vi "NewAndLoad.vi"(0 "EpiWrapper in":refnum<class "EpiWrapper.lvclass">, 1 "StartLotTraveler":T1, 2 "Command":T2=enum."INIT", 3 "error in (no error)":errorcluster, 4 "menu reference":refnum<k9>) -> (5 "EpiWrapper out":refnum<class "EpiWrapper.lvclass">, 6 "Message":string, 7 "error out":errorcluster)   [LabVIEW 2012, in "EpiWrapper.lvclass"]
uses:
  EpiWrapper.lvclass
  Controls/TestType.ctl
  Controls/Command_Enum.ctl
  Controls/StartLotTraveler.ctl
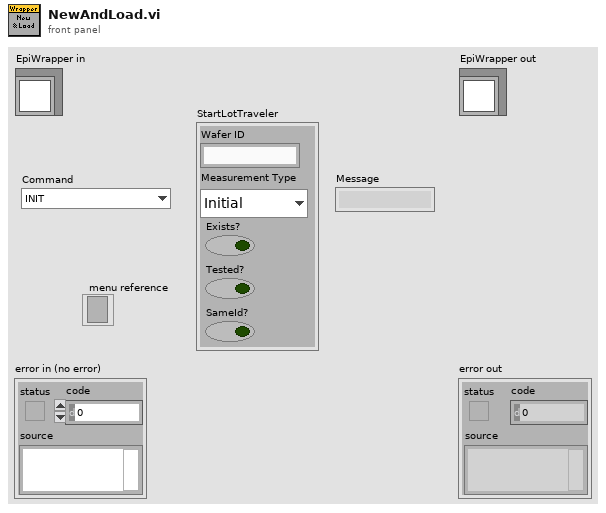
[diagram p1: front panel]
types:
  T1 = typedef "StartLotTraveler.ctl" = cluster{"Wafer ID":string, "Measurement Type":enum16{"Initial", "Final"}, "Exists?":bool, "Tested?":bool, "SameId?":bool}
  T2 = typedef "Command_Enum.ctl" = enum16{"SPECTRUMCAPTURE", "INSITUMEASURE", "RESETCONFIG", "OPENCONFIG", "RESET", "INIT", "LOAD", "MEASURE", "NEW", "SAVE", "UPDATE_INT", "SWAP_MODE", "UPDATE_ACQ", "MARK_MAP_SELECT", "MARK_MAP", "EXIT", "CANCEL"}
  T3 = typedef "TestType.ctl" = string
  T4 = enum8{"Enabled", "Disabled", "Disabled and Grayed Out"}
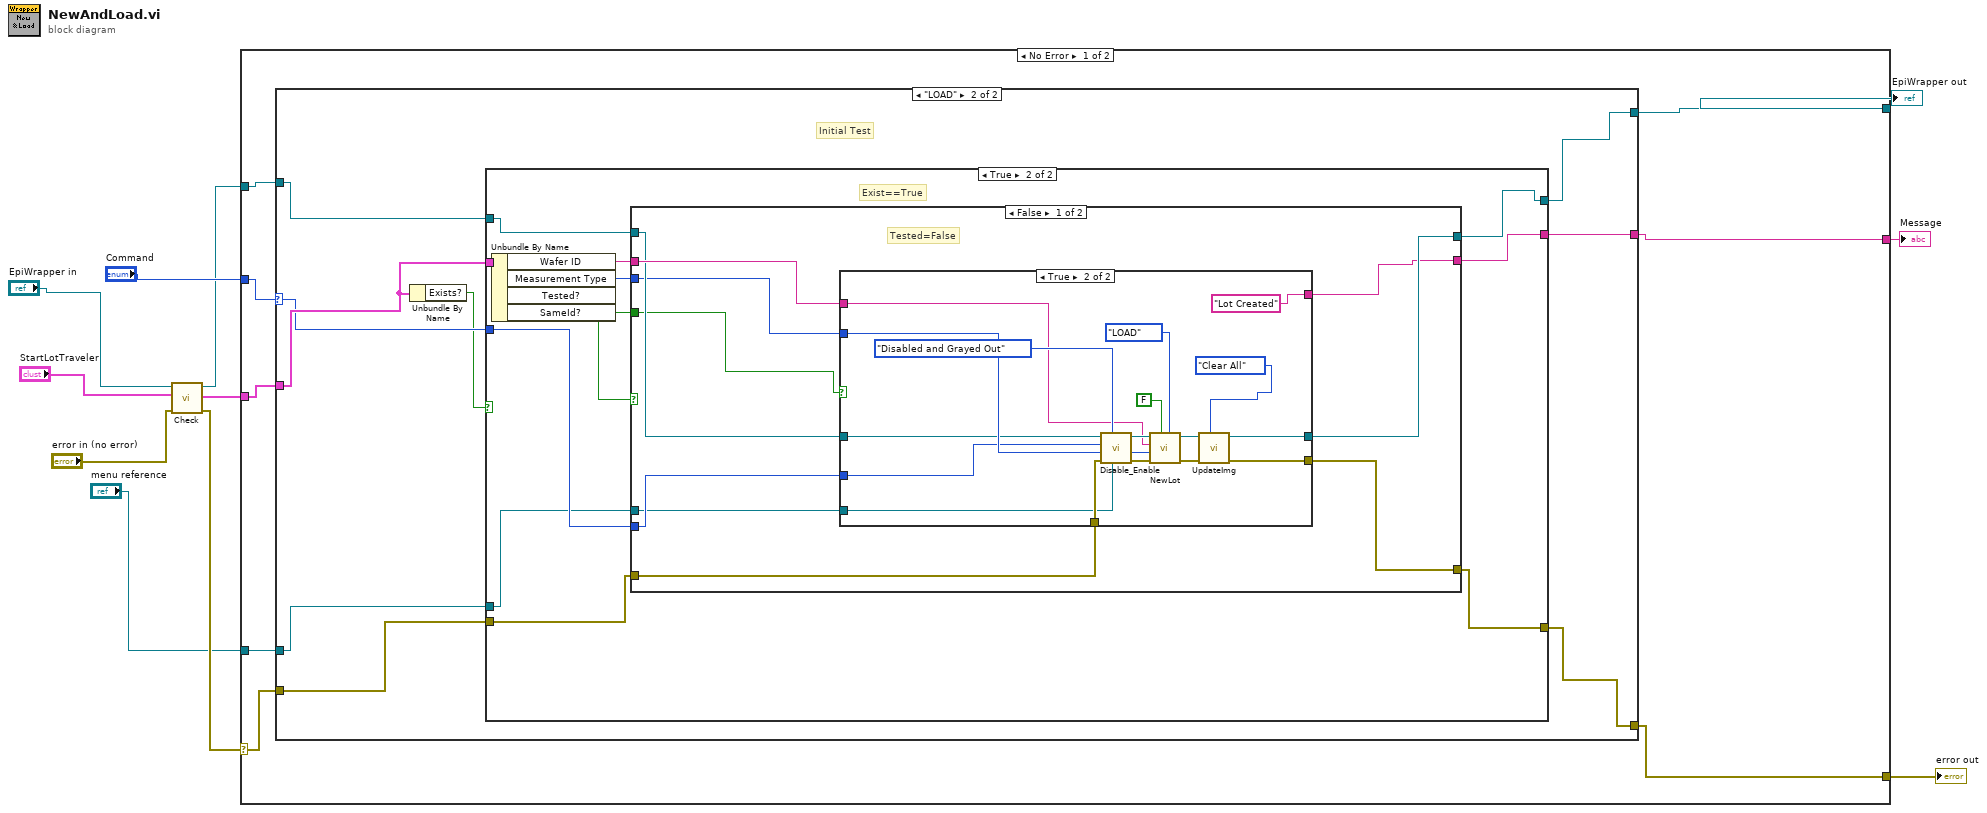
[diagram p0: block diagram]
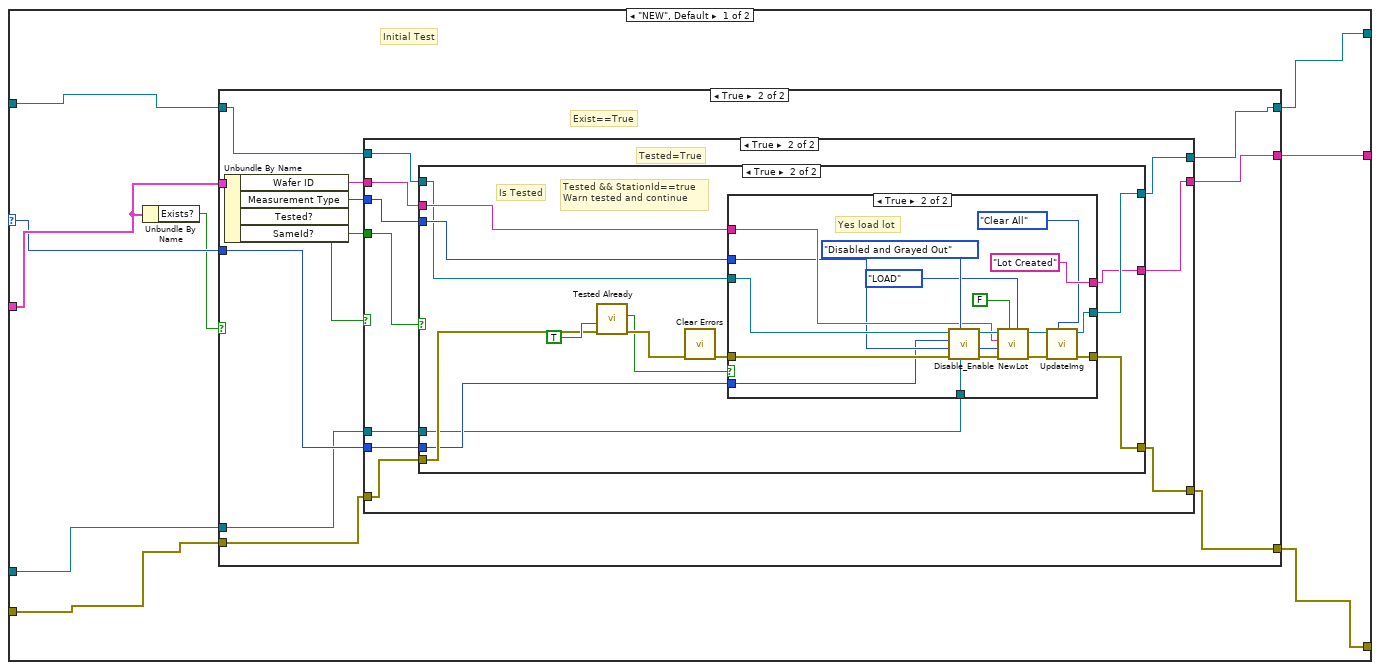
[diagram p2: hidden frame]
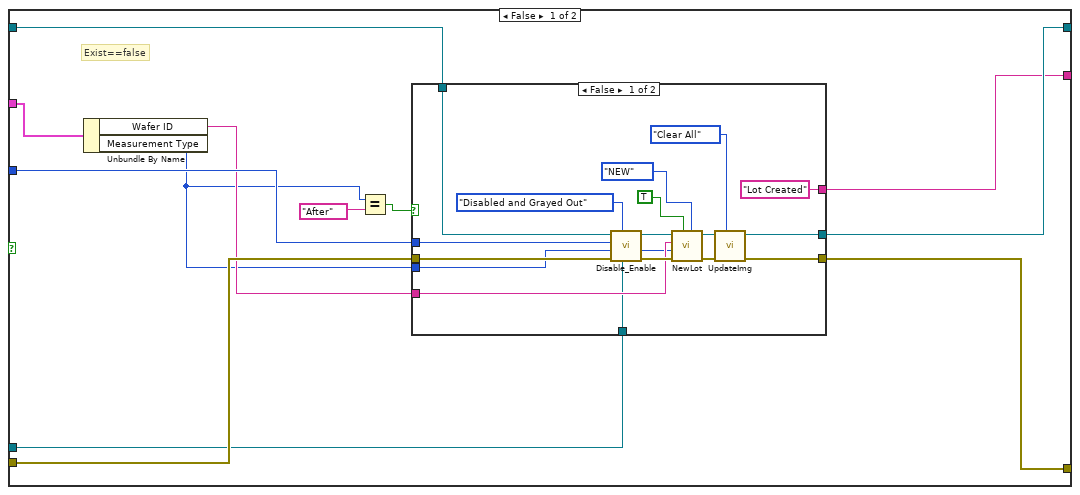
[diagram p3: hidden frame]
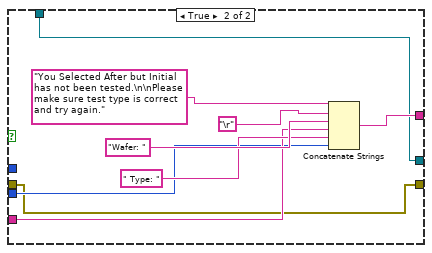
[diagram p4: hidden frame]
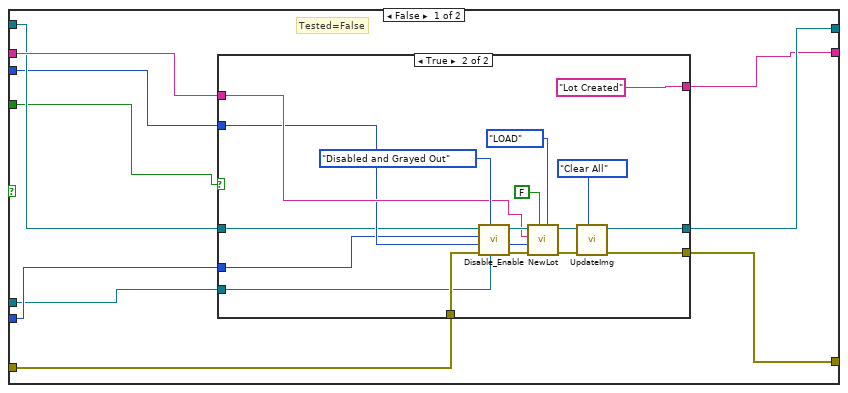
[diagram p5: hidden frame]
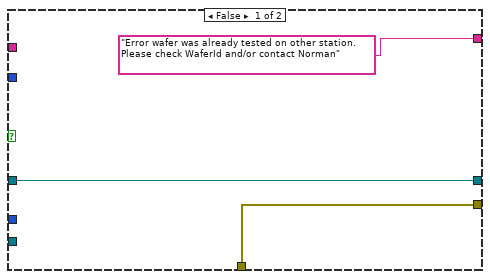
[diagram p6: hidden frame]
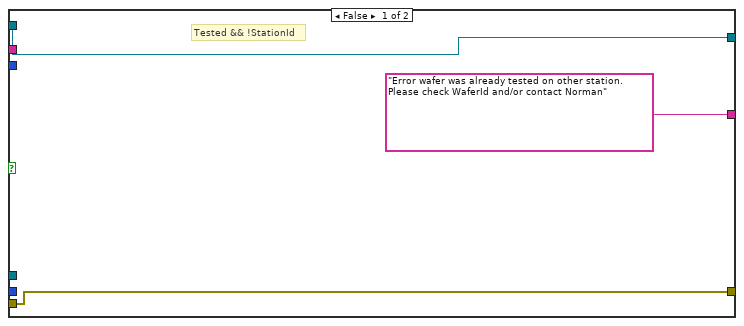
[diagram p7: hidden frame]
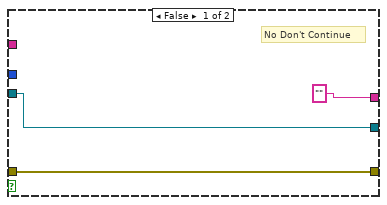
[diagram p8: hidden frame]
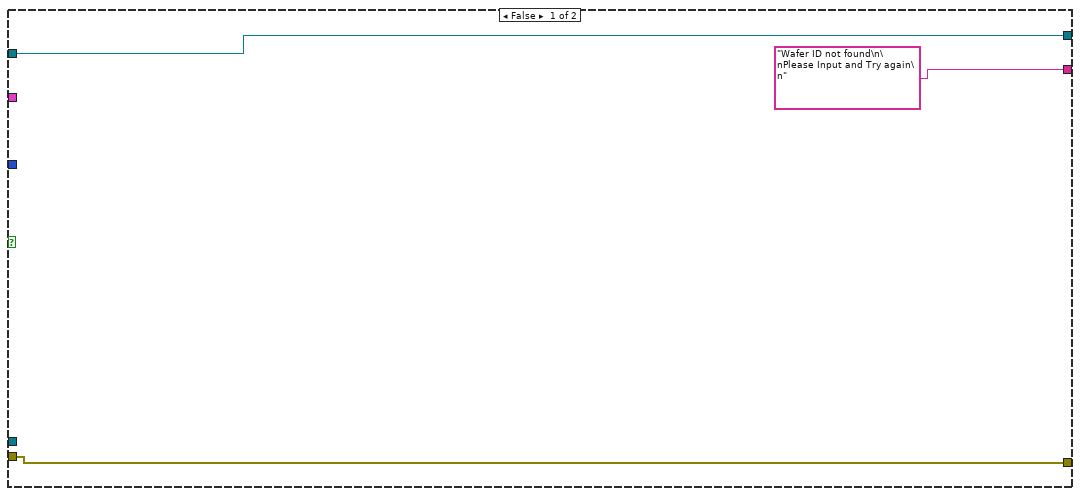
[diagram p9: hidden frame]
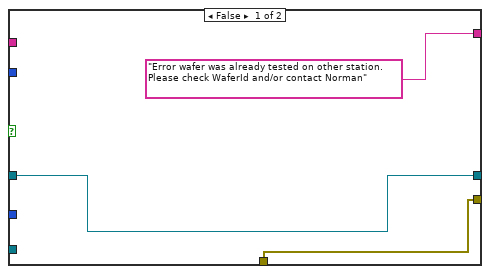
[diagram p10: hidden frame]
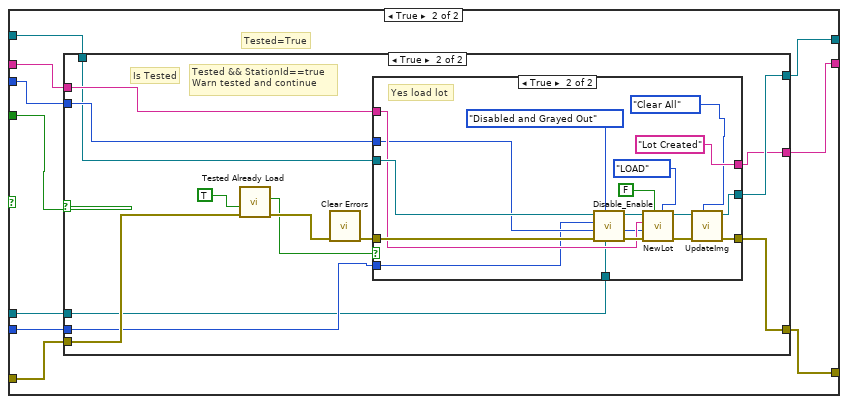
[diagram p11: hidden frame]
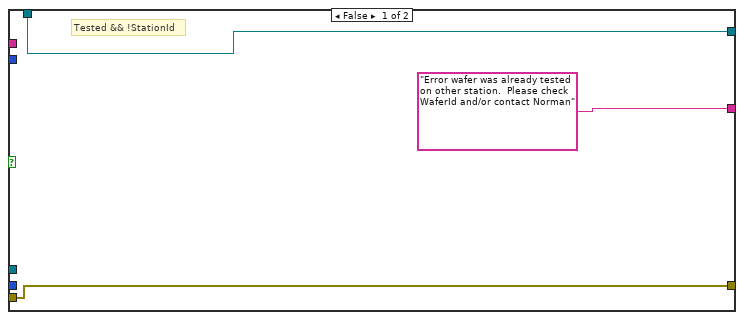
[diagram p12: hidden frame]
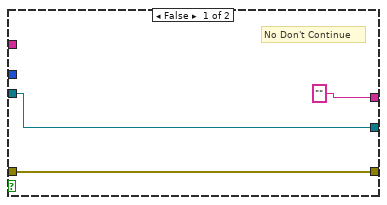
[diagram p13: hidden frame]
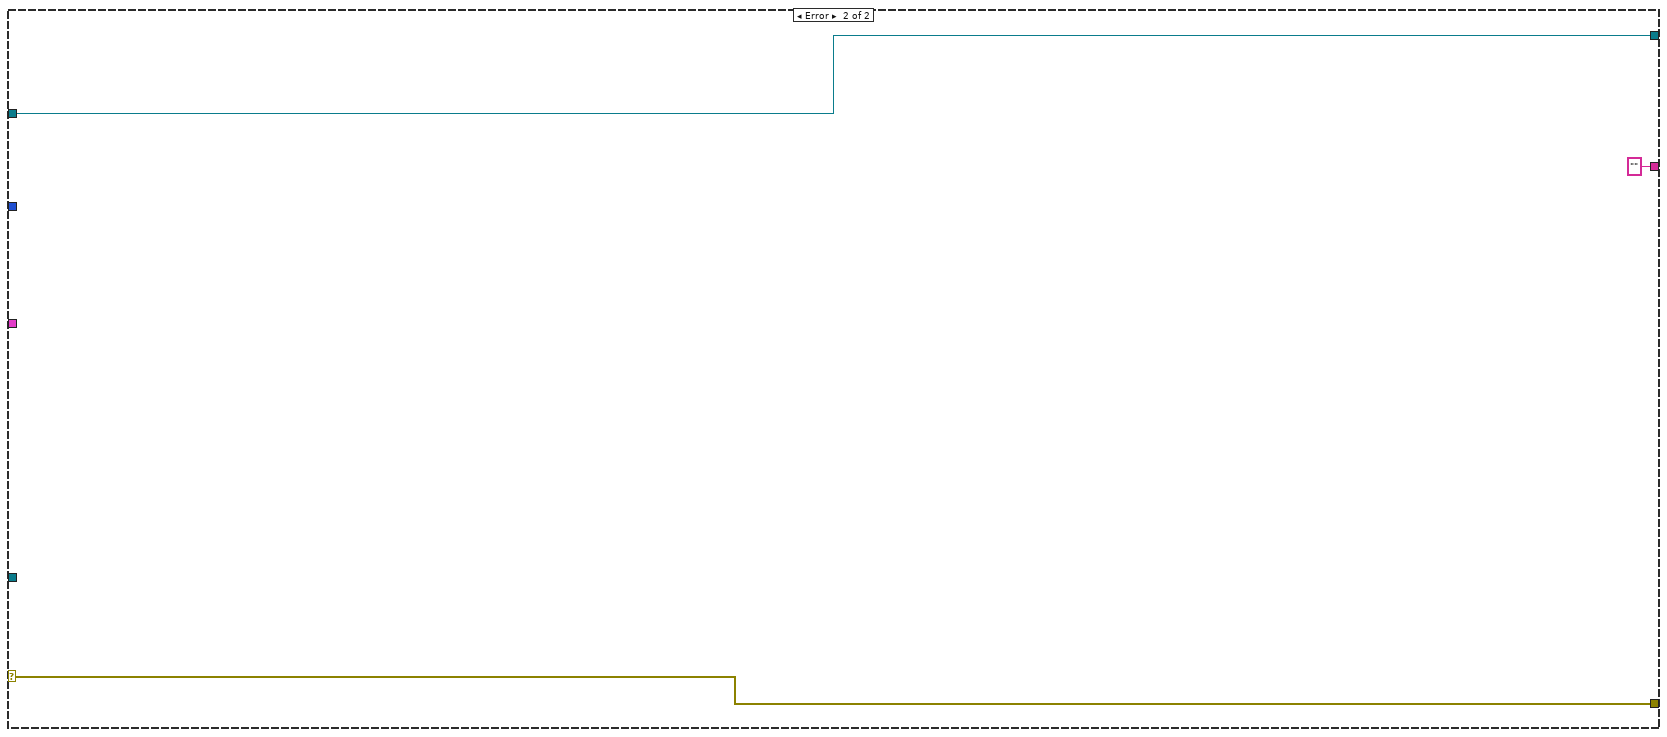
[diagram p14: hidden frame]
diagram:
  n1 = call-dynamic "Check.vi"("error in (no error)"="error in (no error)", "StartLotTraveler In"="StartLotTraveler", "EpiWrapper in"="EpiWrapper in") -> ("error out"=w8:errorcluster, "StartLotTraveler Out"=w7:T1, "EpiWrapper out"=w2:refnum<class "EpiWrapper.lvclass">)  [unwired: 6 in]
  n2 = case shown="No Error" w8 {
    selector: w8 -> [w16 w257]
    tunnel: [w12 w257] -> w11
    tunnel: [w15 w256] -> w10
    tunnel: w2 -> [w17 w256]
    tunnel: w7 -> [w18 _]
    tunnel: "Command" -> [w19 _]
    tunnel: "menu reference" -> [w14 _]
    tunnel: [w13 "" ("x")] -> w1
    frame No Error {
      n3 = case shown="\"LOAD\"" w19 {
        selector: w19 -> [w26 w161]
        tunnel: w18 -> [w28 w163]
        tunnel: w17 -> [w27 w162]
        tunnel: w16 -> [w25 w160]
        tunnel: [w24 w159] -> w15
        tunnel: [w23 w158] -> w12
        tunnel: w14 -> [w22 w157]
        tunnel: [w21 w156] -> w13
        frame "NEW", Default {
          # "Initial Test"
          n4 = Unbundle By Name(w28) -> ("Exists?"=w20:bool)
          n5 = case shown="True" w20 {
            tunnel: w27 -> [w40 w73]
            tunnel: w26 -> [w39 w71]
            tunnel: w25 -> [w38 w72]
            tunnel: w28 -> [w37 w78]
            tunnel: [w35 w68] -> w24
            tunnel: [w34 w69] -> w23
            tunnel: w22 -> [w33 w70]
            tunnel: [w29 w67] -> w21
            frame False {
              # "Exist==false"
              n6 = Unbundle By Name(w37) -> ("Wafer ID"=w36:string, "Measurement Type"=w31:enum16{"Initial", "Final"})
              n7 = Equal?(x=w31, y=T3 "After") -> (x = y?=w30:bool)
              n8 = case shown="False" w30 {
                tunnel: w40 -> [w57 w58]
                tunnel: w39 -> [w56 _]
                tunnel: w38 -> [w55 w59]
                tunnel: w36 -> [w47 w61]
                tunnel: w31 -> [w46 w60]
                tunnel: [w45 w58] -> w35
                tunnel: [w44 w59] -> w34
                tunnel: w33 -> [w43 _]
                tunnel: ["Lot Created" w62] -> w29
                frame False {
                  n9 = call-dynamic "Disable_Enable.vi"("menu reference"=w43, "Disabled"=T4."Disabled and Grayed Out", "error in (no error)"=w55, "Command"=w56, "EpiWrapper in"=w57) -> ("error out"=w51:errorcluster, "EpiWrapper out"=w53:refnum<class "EpiWrapper.lvclass">)  [unwired: 5 in]
                  n10 = call-dynamic "NewLot.vi"("Enum"=enum16{"LOAD", "NEW"}."NEW", "Create Entry?"=TRUE, "error in (no error)"=w51, "Test"=w46, "Wafer ID"=w47, "FrontPanelData in"=w53) -> ("error out"=w52:errorcluster, "FrontPanelData out"=w54:refnum<class "EpiWrapper.lvclass">)  [unwired: 3 in, 1 out]
                  n11 = call-dynamic "UpdateImg.vi"("Enum"=enum16{"Remove", "Mark", "Clear All"}."Clear All", "error in (no error)"=w52, "EpiWrapper in"=w54) -> ("error out"=w44:errorcluster, "EpiWrapper out"=w45:refnum<class "EpiWrapper.lvclass">)  [unwired: 7 in]
                }
                frame True {
                  n12 = Concatenate Strings("You Selected After but Initial has not been tested.\n\nPlease make sure test type is correct and try again.", "\r", "Wafer: " ("string"), w61, " Type: " ("string"), w60) -> (w62:string)
                }
              }
            }
            frame True {
              # "Exist==True"
              n13 = Unbundle By Name(w78) -> ("Wafer ID"=w75:string, "Measurement Type"=w74:enum16{"Initial", "Final"}, "Tested?"=w77:bool, "SameId?"=w76:bool)
              n14 = case shown="True" w77 {
                tunnel: w76 -> [w79 w118]
                tunnel: w75 -> [w88 w117]
                tunnel: w74 -> [w80 w116]
                tunnel: w73 -> [w87 w115]
                tunnel: w72 -> [w85 w114]
                tunnel: w71 -> [w86 w113]
                tunnel: w70 -> [w84 w112]
                tunnel: [w83 w111] -> w69
                tunnel: [w82 w110] -> w68
                tunnel: [w81 w109] -> w67
                frame False {
                  # "Tested=False"
                  n15 = case shown="True" w79 {
                    tunnel: w88 -> [_ w101]
                    tunnel: w80 -> [_ w100]
                    tunnel: w87 -> [w90 w99]
                    tunnel: w86 -> [_ w98]
                    tunnel: w85 -> [w91 w97]
                    tunnel: w84 -> [_ w96]
                    tunnel: [w91 w95] -> w83
                    tunnel: [w90 w94] -> w82
                    tunnel: ["Error wafer was already tested on other station.  Please check WaferId and/or contact Norman" "Lot Created" ("x")] -> w81
                    frame False {
                    }
                    frame True {
                      n16 = call-dynamic "Disable_Enable.vi"("menu reference"=w96, "Disabled"=T4."Disabled and Grayed Out", "error in (no error)"=w97, "Command"=w98, "EpiWrapper in"=w99) -> ("error out"=w107:errorcluster, "EpiWrapper out"=w105:refnum<class "EpiWrapper.lvclass">)  [unwired: 5 in]
                      n17 = call-dynamic "NewLot.vi"("Enum"=enum16{"LOAD", "NEW"}."LOAD", "Create Entry?"=FALSE, "error in (no error)"=w107, "Test"=w100, "Wafer ID"=w101, "FrontPanelData in"=w105) -> ("error out"=w106:errorcluster, "FrontPanelData out"=w104:refnum<class "EpiWrapper.lvclass">)  [unwired: 3 in, 1 out]
                      n18 = call-dynamic "UpdateImg.vi"("Enum"=enum16{"Remove", "Mark", "Clear All"}."Clear All", "error in (no error)"=w106, "EpiWrapper in"=w104) -> ("error out"=w95:errorcluster, "EpiWrapper out"=w94:refnum<class "EpiWrapper.lvclass">)  [unwired: 7 in]
                    }
                  }
                }
                frame True {
                  # "Tested=True"
                  n19 = case shown="True" w118 {
                    tunnel: w117 -> [_ w130]
                    tunnel: w116 -> [_ w129]
                    tunnel: w115 -> [w119 w128]
                    tunnel: w114 -> [w120 w127]
                    tunnel: w113 -> [_ w126]
                    tunnel: w112 -> [_ w125]
                    tunnel: [w120 w124] -> w111
                    tunnel: [w119 w123] -> w110
                    tunnel: ["Error wafer was already tested on other station.  Please check WaferId and/or contact Norman" w122] -> w109
                    frame False {
                      # "Tested && !StationId"
                    }
                    frame True {
                      # "Is Tested"
                      # "Tested && StationId==true\nWarn tested and continue"
                      n20 = call "Tested Already"("error in (no error)"=w127, "Enable"=TRUE) -> ("error out"=w134:errorcluster, "Continue"=w133:bool)  [unwired: 8 in]
                      n21 = call <vilib>:"Clear Errors.vi"("error in (no error)"=w134) -> ("error out"=w131:errorcluster)  [unwired: 6 in]
                      n22 = case shown="True" w133 {
                        tunnel: w131 -> [w137 w153]
                        tunnel: [w137 w150] -> w124
                        tunnel: w128 -> [w136 w146]
                        tunnel: [w136 w145] -> w123
                        tunnel: w130 -> [_ w143]
                        tunnel: w129 -> [_ w142]
                        tunnel: w126 -> [_ w141]
                        tunnel: ["" "Lot Created"] -> w122
                        tunnel: w125 -> [_ w139]
                        frame False {
                          # "No Don't Continue"
                        }
                        frame True {
                          # "Yes load lot"
                          n23 = call-dynamic "Disable_Enable.vi"("menu reference"=w139, "Disabled"=T4."Disabled and Grayed Out", "error in (no error)"=w153, "Command"=w141, "EpiWrapper in"=w146) -> ("error out"=w152:errorcluster, "EpiWrapper out"=w147:refnum<class "EpiWrapper.lvclass">)  [unwired: 5 in]
                          n24 = call-dynamic "NewLot.vi"("Enum"=enum16{"LOAD", "NEW"}."LOAD", "Create Entry?"=FALSE, "error in (no error)"=w152, "Test"=w142, "Wafer ID"=w143, "FrontPanelData in"=w147) -> ("error out"=w151:errorcluster, "FrontPanelData out"=w148:refnum<class "EpiWrapper.lvclass">)  [unwired: 3 in, 1 out]
                          n25 = call-dynamic "UpdateImg.vi"("Enum"=enum16{"Remove", "Mark", "Clear All"}."Clear All", "error in (no error)"=w151, "EpiWrapper in"=w148) -> ("error out"=w150:errorcluster, "EpiWrapper out"=w145:refnum<class "EpiWrapper.lvclass">)  [unwired: 7 in]
                        }
                      }
                    }
                  }
                }
              }
            }
          }
        }
        frame "LOAD" {
          # "Initial Test"
          n26 = Unbundle By Name(w163) -> ("Exists?"=w155:bool)
          n27 = case shown="True" w155 {
            tunnel: w162 -> [w165 w173]
            tunnel: w161 -> [_ w171]
            tunnel: w160 -> [w164 w172]
            tunnel: w163 -> [_ w178]
            tunnel: [w165 w168] -> w159
            tunnel: [w164 w169] -> w158
            tunnel: w157 -> [_ w170]
            tunnel: ["Wafer ID not found\n\nPlease Input and Try again\n" w167] -> w156
            frame False {
            }
            frame True {
              # "Exist==True"
              n28 = Unbundle By Name(w178) -> ("Wafer ID"=w175:string, "Measurement Type"=w174:enum16{"Initial", "Final"}, "Tested?"=w177:bool, "SameId?"=w176:bool)
              n29 = case shown="False" w177 {
                tunnel: w176 -> [w179 w209]
                tunnel: w175 -> [w188 w218]
                tunnel: w174 -> [w181 w217]
                tunnel: w173 -> [w187 w216]
                tunnel: w172 -> [w185 w215]
                tunnel: w171 -> [w186 w214]
                tunnel: w170 -> [w184 w213]
                tunnel: [w183 w212] -> w169
                tunnel: [w182 w211] -> w168
                tunnel: [w180 w210] -> w167
                frame False {
                  # "Tested=False"
                  n30 = case shown="True" w179 {
                    tunnel: w188 -> [_ w201]
                    tunnel: w181 -> [_ w200]
                    tunnel: w187 -> [w190 w199]
                    tunnel: w186 -> [_ w198]
                    tunnel: w185 -> [w191 w197]
                    tunnel: w184 -> [_ w196]
                    tunnel: [w191 w195] -> w183
                    tunnel: [w190 w194] -> w182
                    tunnel: ["Error wafer was already tested on other station.  Please check WaferId and/or contact Norman" "Lot Created" ("x")] -> w180
                    frame False {
                    }
                    frame True {
                      n31 = call-dynamic "Disable_Enable.vi"("menu reference"=w196, "Disabled"=T4."Disabled and Grayed Out", "error in (no error)"=w197, "Command"=w198, "EpiWrapper in"=w199) -> ("error out"=w207:errorcluster, "EpiWrapper out"=w205:refnum<class "EpiWrapper.lvclass">)  [unwired: 5 in]
                      n32 = call-dynamic "NewLot.vi"("Enum"=enum16{"LOAD", "NEW"}."LOAD", "Create Entry?"=FALSE, "error in (no error)"=w207, "Test"=w200, "Wafer ID"=w201, "FrontPanelData in"=w205) -> ("error out"=w206:errorcluster, "FrontPanelData out"=w204:refnum<class "EpiWrapper.lvclass">)  [unwired: 3 in, 1 out]
                      n33 = call-dynamic "UpdateImg.vi"("Enum"=enum16{"Remove", "Mark", "Clear All"}."Clear All", "error in (no error)"=w206, "EpiWrapper in"=w204) -> ("error out"=w195:errorcluster, "EpiWrapper out"=w194:refnum<class "EpiWrapper.lvclass">)  [unwired: 7 in]
                    }
                  }
                }
                frame True {
                  # "Tested=True"
                  n34 = case shown="True" w209 {
                    tunnel: w218 -> [_ w230]
                    tunnel: w217 -> [_ w229]
                    tunnel: w216 -> [w219 w228]
                    tunnel: w215 -> [w220 w227]
                    tunnel: w214 -> [_ w226]
                    tunnel: w213 -> [_ w225]
                    tunnel: [w220 w224] -> w212
                    tunnel: [w219 w223] -> w211
                    tunnel: ["Error wafer was already tested on other station.  Please check WaferId and/or contact Norman" w222] -> w210
                    frame False {
                      # "Tested && !StationId"
                    }
                    frame True {
                      # "Is Tested"
                      # "Tested && StationId==true\nWarn tested and continue"
                      n35 = call "Tested Already Load"("error in (no error)"=w227, "Enable"=TRUE) -> ("error out"=w234:errorcluster, "Continue"=w233:bool)  [unwired: 8 in]
                      n36 = call <vilib>:"Clear Errors.vi"("error in (no error)"=w234) -> ("error out"=w231:errorcluster)  [unwired: 6 in]
                      n37 = case shown="True" w233 {
                        tunnel: w231 -> [w237 w253]
                        tunnel: [w237 w250] -> w224
                        tunnel: w228 -> [w236 w246]
                        tunnel: [w236 w245] -> w223
                        tunnel: w230 -> [_ w243]
                        tunnel: w229 -> [_ w242]
                        tunnel: w226 -> [_ w241]
                        tunnel: ["" "Lot Created"] -> w222
                        tunnel: w225 -> [_ w239]
                        frame False {
                          # "No Don't Continue"
                        }
                        frame True {
                          # "Yes load lot"
                          n38 = call-dynamic "Disable_Enable.vi"("menu reference"=w239, "Disabled"=T4."Disabled and Grayed Out", "error in (no error)"=w253, "Command"=w241, "EpiWrapper in"=w246) -> ("error out"=w252:errorcluster, "EpiWrapper out"=w247:refnum<class "EpiWrapper.lvclass">)  [unwired: 5 in]
                          n39 = call-dynamic "NewLot.vi"("Enum"=enum16{"LOAD", "NEW"}."LOAD", "Create Entry?"=FALSE, "error in (no error)"=w252, "Test"=w242, "Wafer ID"=w243, "FrontPanelData in"=w247) -> ("error out"=w251:errorcluster, "FrontPanelData out"=w248:refnum<class "EpiWrapper.lvclass">)  [unwired: 3 in, 1 out]
                          n40 = call-dynamic "UpdateImg.vi"("Enum"=enum16{"Remove", "Mark", "Clear All"}."Clear All", "error in (no error)"=w251, "EpiWrapper in"=w248) -> ("error out"=w250:errorcluster, "EpiWrapper out"=w245:refnum<class "EpiWrapper.lvclass">)  [unwired: 7 in]
                        }
                      }
                    }
                  }
                }
              }
            }
          }
        }
      }
    }
    frame Error {
    }
  }
  "error out" <- w11
  "EpiWrapper out" <- w10
  "Message" <- w1
